vi "Voltage Update.vi"(8 "error in (no error)":errorcluster, 9 "Amplifier Gain":dbl=1.0 min=-15.0 max=15.0, 10 "Voltage Output":dbl(slide) min=-50.0 max=50.0 scale=-45.0..45.0, 11 "Physical Channel":tag="Dev2/ao0") -> (0 "error out":errorcluster, 2 "DAQ output":dbl(slide)=-0.0 min=-3.5 max=3.5 scale=-3.5..3.5)   [LabVIEW 2016, in "Transport.lvclass"]
doc: "I. Description:\nThis example demonstrates how to output a single Voltage Update (Sample) to an Analog Output Channel.\n\nII. Instructions for Running:\n1. Select the Physical Channel to correspond to where your signal is output on the DAQ device.\n2. Enter the Minimum and Maximum Voltage Ranges\nNote: Use the Acq One Sample example to verify you are generating the correct output on the DAQ device\n\nIII. Block Diagram Steps:\n1. Create an Analog Output Voltage Channel\n2. Use the Write VI to Output 1 Sample to 1 Channel on the Data\nAcquisition Card. \n3. Call the Clear Task VI to clear the Task.\n4. Use the popup dialog box to display an error if any. \n\nIV. I/O Connections Overview:\nMake sure your signal output terminal matches the Physical Channel I/O Control. For further connection information, refer to your hardware reference manual."
uses:
  Transport.lvclass
  <vilib>/DAQmx/write.llb/DAQmx Write (Analog 1D DBL 1Chan NSamp).vi
  <vilib>/DAQmx/write.llb/DAQmx Write (Analog DBL 1Chan 1Samp).vi
  <vilib>/DAQmx/create/channels.llb/DAQmx Create Channel (AO-Voltage-Basic).vi
  <vilib>/DAQmx/configure/timing.llb/DAQmx Timing (Sample Clock).vi
  <vilib>/DAQmx/miscellaneous.llb/DAQmx Fill In Error Info.vi
  <resource>/objmgr/daqmx.rc
panel:
  in  "Maximum Value":dbl=3.5
  in  "Minimum Value":dbl=-3.5 min=-3.5 max=0.0
  # "Waveform Settings"
  # "Channel Settings"
  # "Instructions"
  # "-This VI will set a DC output to a NI USB-4431 DSA DAQ\n-The absolute limits are +/- 3.5 V\n- The voltage will be maintained even when the VI is not running & if LabVIEW is shutdown"
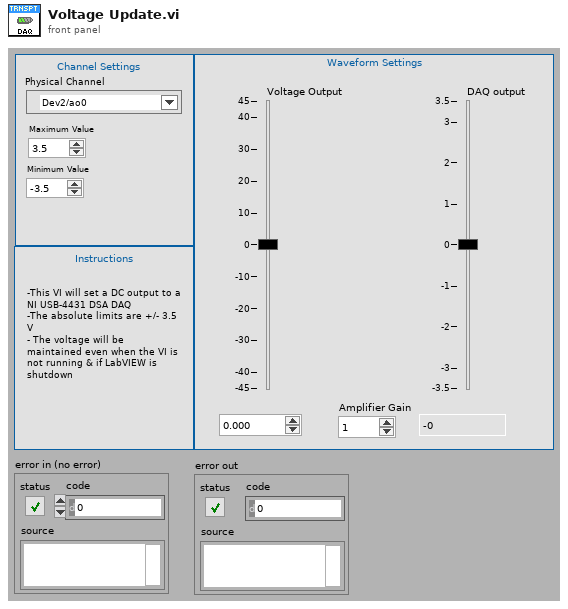
[diagram p1: front panel]
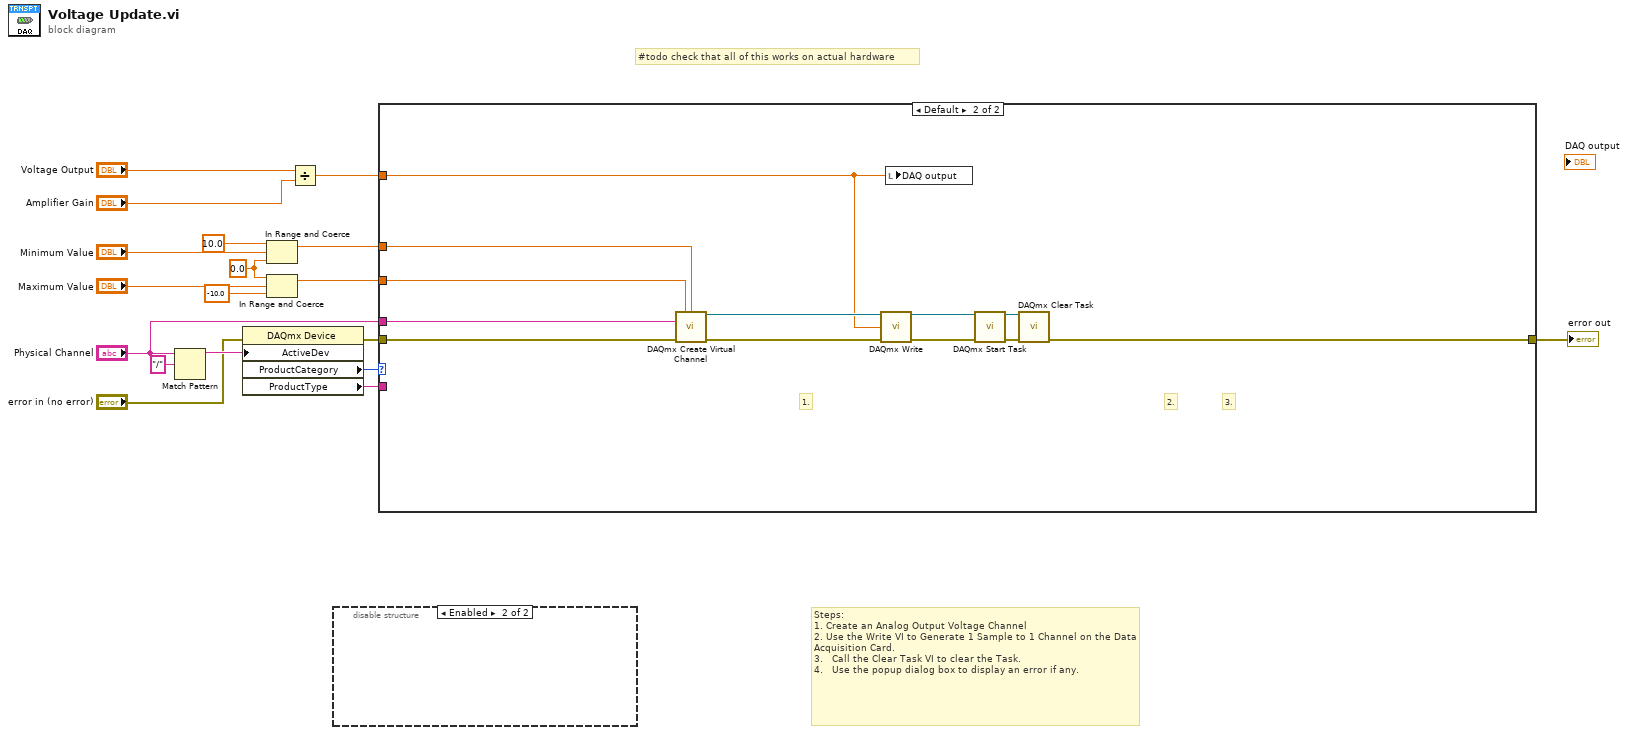
[diagram p0: block diagram]
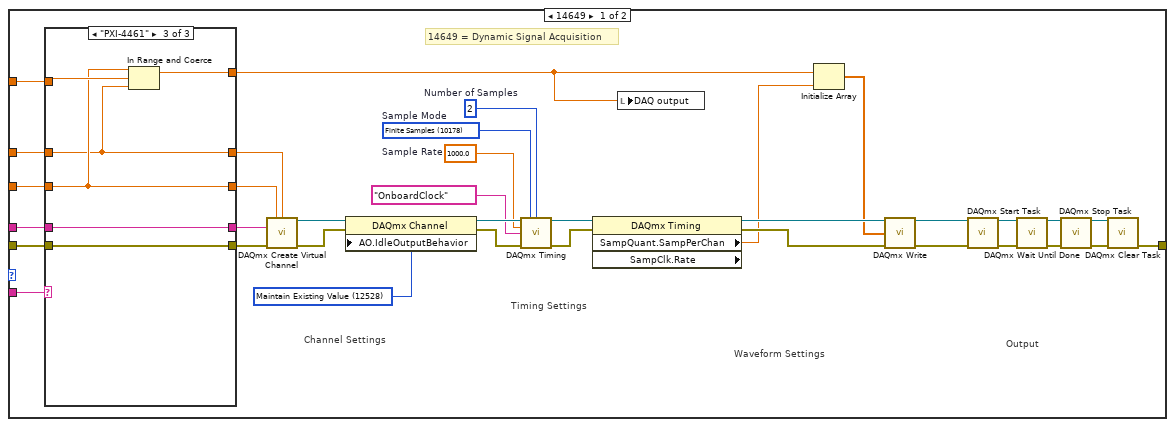
[diagram p2: hidden frame]
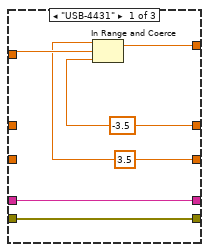
[diagram p3: hidden frame]
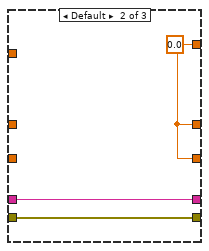
[diagram p4: hidden frame]
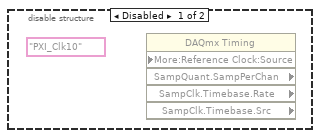
[diagram p5: hidden frame]
diagram:
  w1 = 0.0 ("upper limit")
  # "#todo check that all of this works on actual hardware"
  # "Steps: \n1. Create an Analog Output Voltage Channel\n2. Use the Write VI to Generate 1 Sample to 1 Channel on the Data Acquisition Card.  \n3.   Call the Clear Task VI to clear the Task.\n4.   Use the popup dialog box to display an error if any."
  n1 = Match Pattern(string="Physical Channel", regular expression="/") -> (before substring=w16:string)  [unwired: 1 in, 3 out]
  n2 = property class="DAQmx Device"(error in="error in (no error)", "ActiveDev"=w16) -> (error out=w15:errorcluster, "ProductCategory"=w13:i32, "ProductType"=w11:string)  [unwired: 1 in, 1 out]
  n3 = In Range and Coerce(upper limit=10.0, x="Minimum Value", lower limit=w1) -> (coerced(x)=w3:dbl)  [unwired: 1 out]
  n4 = In Range and Coerce(upper limit=w1, x="Maximum Value", lower limit=-10.0) -> (coerced(x)=w2:dbl)  [unwired: 1 out]
  n5 = Divide(x="Voltage Output", y="Amplifier Gain") -> (x/y=w12:dbl)
  n6 = disable-structure shown="Enabled" {
    frame Disabled {
      (unwired) tag "PXI_Clk10" ("RefClk.Src")
      n7 = property class="DAQmx Timing" props=["More:Reference Clock:Source", "SampQuant.SampPerChan", "SampClk.Timebase.Rate", "SampClk.Timebase.Src"]() -> ()  [unwired: 3 in, 5 out]
    }
    frame Enabled {
    }
  }
  n8 = case shown="Default" w13 {
    tunnel: [w22 w80] -> w18
    tunnel: w15 -> [w23 w73]
    tunnel: "Physical Channel" -> [w26 w72]
    tunnel: w12 -> [w27 w69]
    tunnel: w11 -> [w53 _]
    tunnel: w2 -> [w30 w71]
    tunnel: w3 -> [w28 w70]
    frame 14649 {
      w42 = 2  # Number of Samples
      w36 = 1000.0  # Sample Rate
      w50 = 12528 items=["Zero Volts"=12526, "High-Impedance"=12527, "Maintain Existing Value"=12528] ("AO.IdleOutputBehavior")
      w33 = 10178 items=["Finite Samples"=10178, "Continuous Samples"=10123, "Hardware Timed Single Point"=12522]  # Sample Mode
      # "Output"
      # "Waveform Settings"
      # "Timing Settings"
      # "Channel Settings"
      # "14649 = Dynamic Signal Acquisition"
      n9 = case shown="\"PXI-4461\"" w53 {
        tunnel: [w58 w62 w66] -> w31
        tunnel: w30 -> [_ _ w66]
        tunnel: [w57 w62 w65] -> w29
        tunnel: w28 -> [_ _ w65]
        tunnel: w27 -> [w59 _ w68]
        tunnel: [w56 w62 w67] -> w20
        tunnel: w26 -> [w55 w60 w63]
        tunnel: [w55 w60 w63] -> w25
        tunnel: [w54 w61 w64] -> w24
        tunnel: w23 -> [w54 w61 w64]
        frame "USB-4431" {
          w58 = 3.5 ("Maximum Value")
          w57 = -3.5 ("Minimum Value")
          n10 = In Range and Coerce(upper limit=w58, x=w59, lower limit=w57) -> (coerced(x)=w56:dbl)  [unwired: 1 out]
        }
        frame Default {
          w62 = 0.0 ("Maximum Value")
        }
        frame "PXI-4461" {
          n11 = In Range and Coerce(upper limit=w66, x=w68, lower limit=w65) -> (coerced(x)=w67:dbl)  [unwired: 1 out]
        }
      }
      n12 = call-poly <vilib>:"DAQmx Create Virtual Channel.vi"("maximum value"=w31, "minimum value"=w29, "physical channels"=w25, "error in"=w24) -> ("task out"=w34:refnum<k21>, "error out"=w48:errorcluster)  [unwired: 10 in]
      n13 = property class="DAQmx Channel"(reference=w34, error in=w48, "AO.IdleOutputBehavior"=w50) -> (reference out=w47:refnum<k21>, error out=w49:errorcluster)
      n14 = call-poly <vilib>:"DAQmx Timing.vi"("task/channels in"=w47, "sample mode"=w33, "samples per channel"=w42, "rate"=w36, "source"=tag "OnboardClock" ("Sample Clock Source"), "error in"=w49) -> ("task out"=w32:refnum<k21>, "error out"=w52:errorcluster)  [unwired: 8 in]
      n15 = property class="DAQmx Timing" props=["SampQuant.SampPerChan", "SampClk.Rate"](reference=w32, error in=w52) -> (reference out=w37:refnum<k21>, error out=w51:errorcluster, "SampQuant.SampPerChan"=w21:dbl)  [unwired: 1 out]
      n16 = local write "DAQ output"(w20) -> ()
      n17 = Initialize Array(w20, w21) -> (w19:dbl[])
      n18 = call-poly <vilib>:"DAQmx Write.vi"("task/channels in"=w37, "data"=w19, "error in"=w51) -> ("task out"=w38:refnum<k21>, "error out"=w39:errorcluster)  [unwired: 10 in, 1 out]
      n19 = call <vilib>:"DAQmx Start Task.vi"("task/channels in"=w38, "error in"=w39) -> ("task out"=w40:refnum<k21>, "error out"=w41:errorcluster)  [unwired: 12 in]
      n20 = call <vilib>:"DAQmx Wait Until Done.vi"("task/channels in"=w40, "error in"=w41) -> ("task out"=w45:refnum<k21>, "error out"=w46:errorcluster)  [unwired: 12 in]
      n21 = call <vilib>:"DAQmx Stop Task.vi"("task/channels in"=w45, "error in"=w46) -> ("task out"=w43:refnum<k21>, "error out"=w44:errorcluster)  [unwired: 12 in]
      n22 = call <vilib>:"DAQmx Clear Task.vi"("task in"=w43, "error in"=w44) -> ("error out"=w22:errorcluster)  [unwired: 13 in]
    }
    frame Default {
      # "2."
      # "3."
      # "1."
      n23 = call-poly <vilib>:"DAQmx Create Virtual Channel.vi"("maximum value"=w71, "minimum value"=w70, "physical channels"=w72, "error in"=w73) -> ("task out"=w79:refnum<k21>, "error out"=w78:errorcluster)  [unwired: 10 in]
      n24 = call-poly <vilib>:"DAQmx Write.vi"("task/channels in"=w79, "data"=w69, "error in"=w78) -> ("task out"=w74:refnum<k21>, "error out"=w75:errorcluster)  [unwired: 10 in, 1 out]
      n25 = local write "DAQ output"(w69) -> ()
      n26 = call <vilib>:"DAQmx Start Task.vi"("task/channels in"=w74, "error in"=w75) -> ("task out"=w77:refnum<k21>, "error out"=w76:errorcluster)  [unwired: 12 in]
      n27 = call <vilib>:"DAQmx Clear Task.vi"("task in"=w77, "error in"=w76) -> ("error out"=w80:errorcluster)  [unwired: 13 in]
    }
  }
  "error out" <- w18
